vi "nocsac_iface.vi"() -> ()   [LabVIEW 2011]
uses:
  Globals.vi
panel:
  out "Enum":enum16{""}(ring)
  in  "Unlock Door":bool
  out "Door state":bool
  in  "Tab Control":enum32{"Config", "Diag"}(tab)
  in  "Net":bool
  in  "Monitor":i32
  in  "Port":u16
  in  "Node ID":dbl
  out "Conn":bool
  out "remote address":string
  out "remote port":u16
  out "Node ID":u32
  out "Input?":bool
  out "Output?":bool
  out "Psi":bool
  out "Chi":bool
  out "Phi":bool
  out "Upsilon":bool
  out "Omega":bool
  out "Tau":bool
  out "Rho":bool
  out "Pi":bool
  out "Omicron":bool
  out "Xi":bool
  out "Sigma":bool
  out "Nu":bool
  out "Lambda":bool
  out "Kappa":bool
  out "Iota":bool
  out "Theta":bool
  out "Mu":bool
  out "Eta":bool
  out "Epsilon":bool
  out "Delta":bool
  out "Gamma":bool
  out "Beta":bool
  out "Zeta":bool
  out "Alpha":bool
  in  "OMEGA":bool
  in  "PSI":bool
  in  "CHI":bool
  in  "PHI":bool
  in  "UPSILON":bool
  in  "TAU":bool
  in  "SIGMA":bool
  in  "RHO":bool
  in  "PI":bool
  in  "OMICRON":bool
  in  "XI":bool
  in  "NU":bool
  in  "MU":bool
  in  "LAMBDA":bool
  in  "KAPPA":bool
  in  "IOTA":bool
  in  "THETA":bool
  in  "ETA":bool
  in  "ZETA":bool
  in  "EPSILON":bool
  in  "DELTA":bool
  in  "GAMMA":bool
  in  "BETA":bool
  in  "ALPHA":bool
  in  "stop":bool
  in  "Orange":bool
  in  "Chartreuse":bool
  in  "Green":bool
  in  "Fuchsia":bool
  in  "Black":bool
  in  "Grey":bool
  in  "Vermillion":bool
  in  "Beige":bool
  in  "Gold":bool
  in  "Yellow":bool
  in  "Blue":bool
  in  "Red":bool
  out "Red":bool
  out "Orange":bool
  out "Yellow":bool
  out "Green":bool
  out "Vermillion":bool
  out "Orange":bool
  out "Chartreuse":bool
  out "Green":bool
  out "Fuchsia":bool
  out "Black":bool
  out "Grey":bool
  out "Beige":bool
  out "Gold":bool
  out "Yellow":bool
  out "Blue":bool
  out "Red":bool
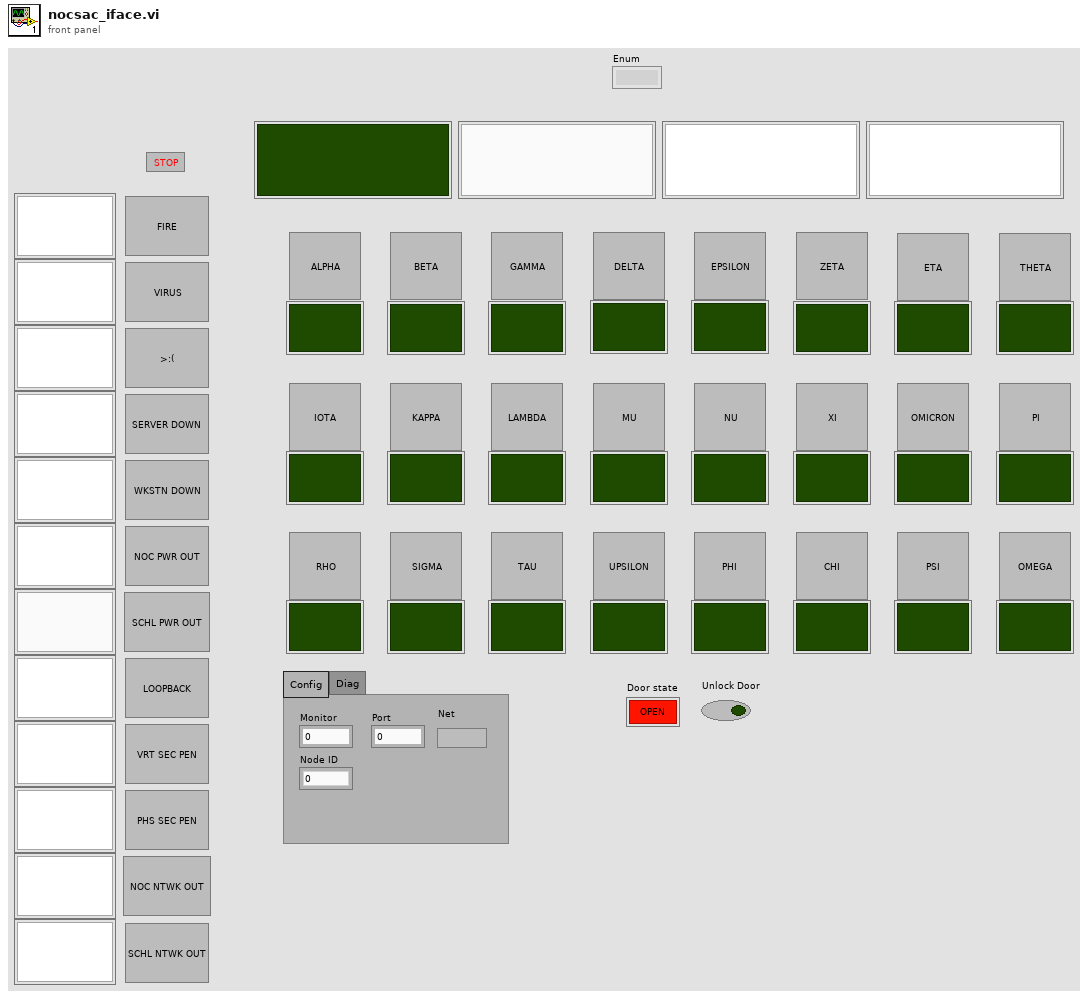
[diagram p1: front panel]
types:
  T1 = typedef "LVAllMonitorsDisplayTypeDef.ctl" = cluster{"Bounds":cluster{"Left":i16, "Top":i16, "Right":i16, "Bottom":i16}, "Depth":i16}[]
  T2 = cluster{"Alpha":bool, "Beta":bool, "Gamma":bool, "Delta":bool, "Epsilon":bool, "Zeta":bool, "Eta":bool, "Theta":bool, "Iota":bool, "Kappa":bool, "Lambda":bool, "Mu":bool, "Nu":bool, "Xi":bool, "Omicron":bool, "Pi":bool, "Rho":bool, "Sigma":bool, "Tau":bool, "Upsilon":bool, "Phi":bool, "Chi":bool, "Psi":bool, "Omega":bool}
  T3 = cluster{"Red":bool, "Blue":bool, "Yellow":bool, "Gold":bool, "Beige":bool, "Grey":bool, "Black":bool, "Fuchsia":bool, "Green":bool, "Chartreuse":bool, "Orange":bool, "Vermillion":bool}
  T4 = cluster{"Bounds":cluster{"Left":i16, "Top":i16, "Right":i16, "Bottom":i16}, "Depth":i16}
  T5 = cluster{"Left":i16, "Top":i16, "Right":i16, "Bottom":i16}
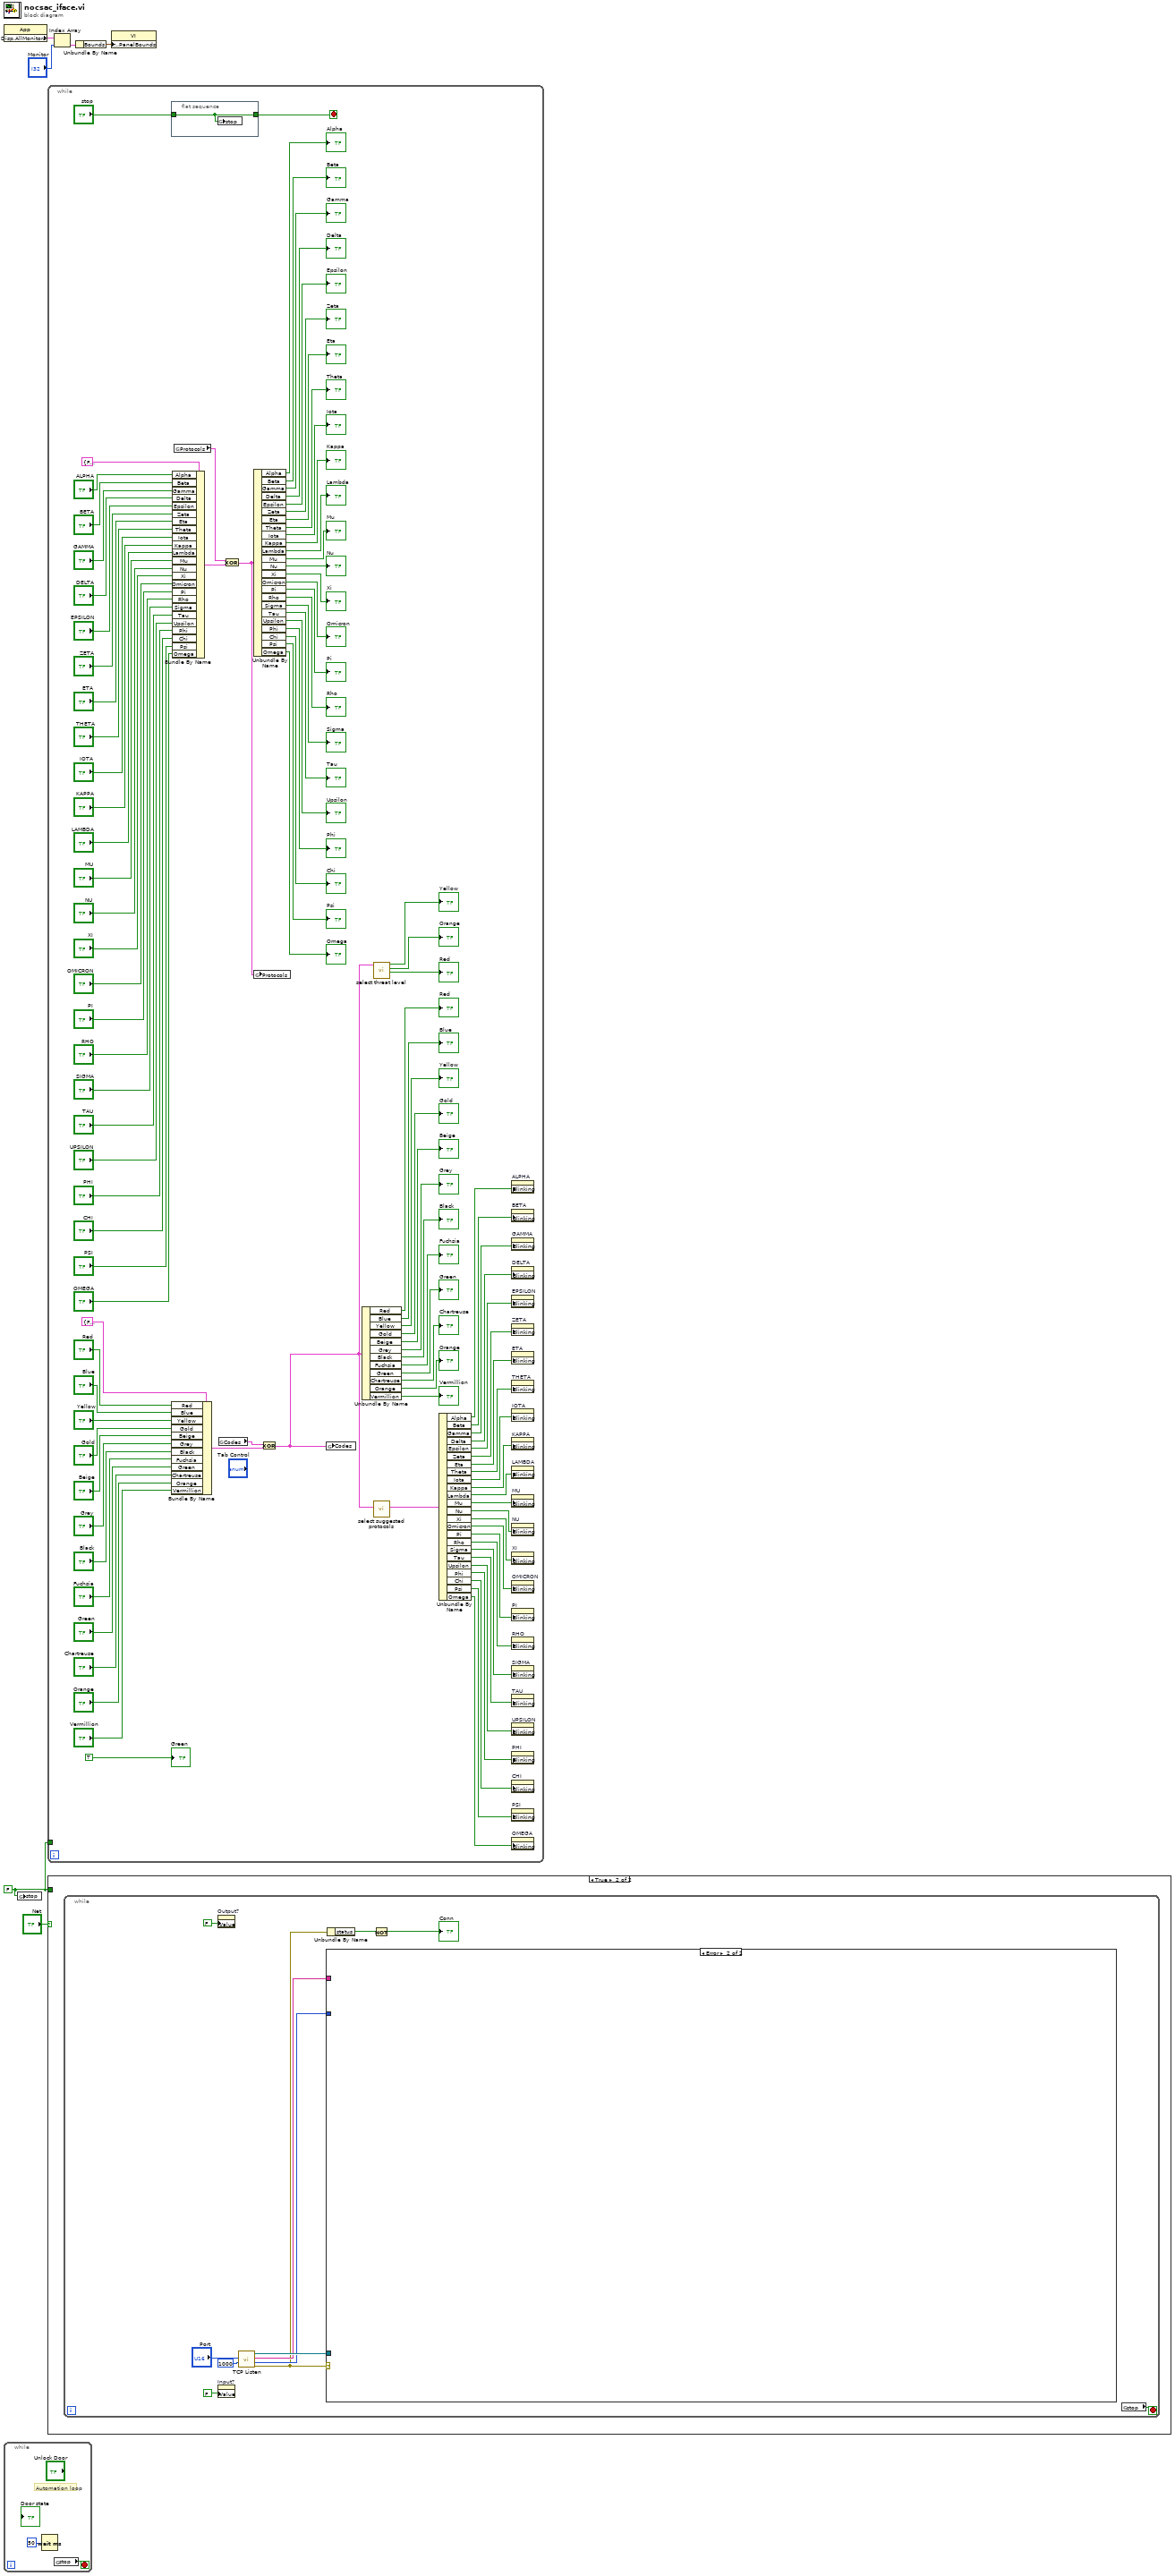
[diagram p0: block diagram]
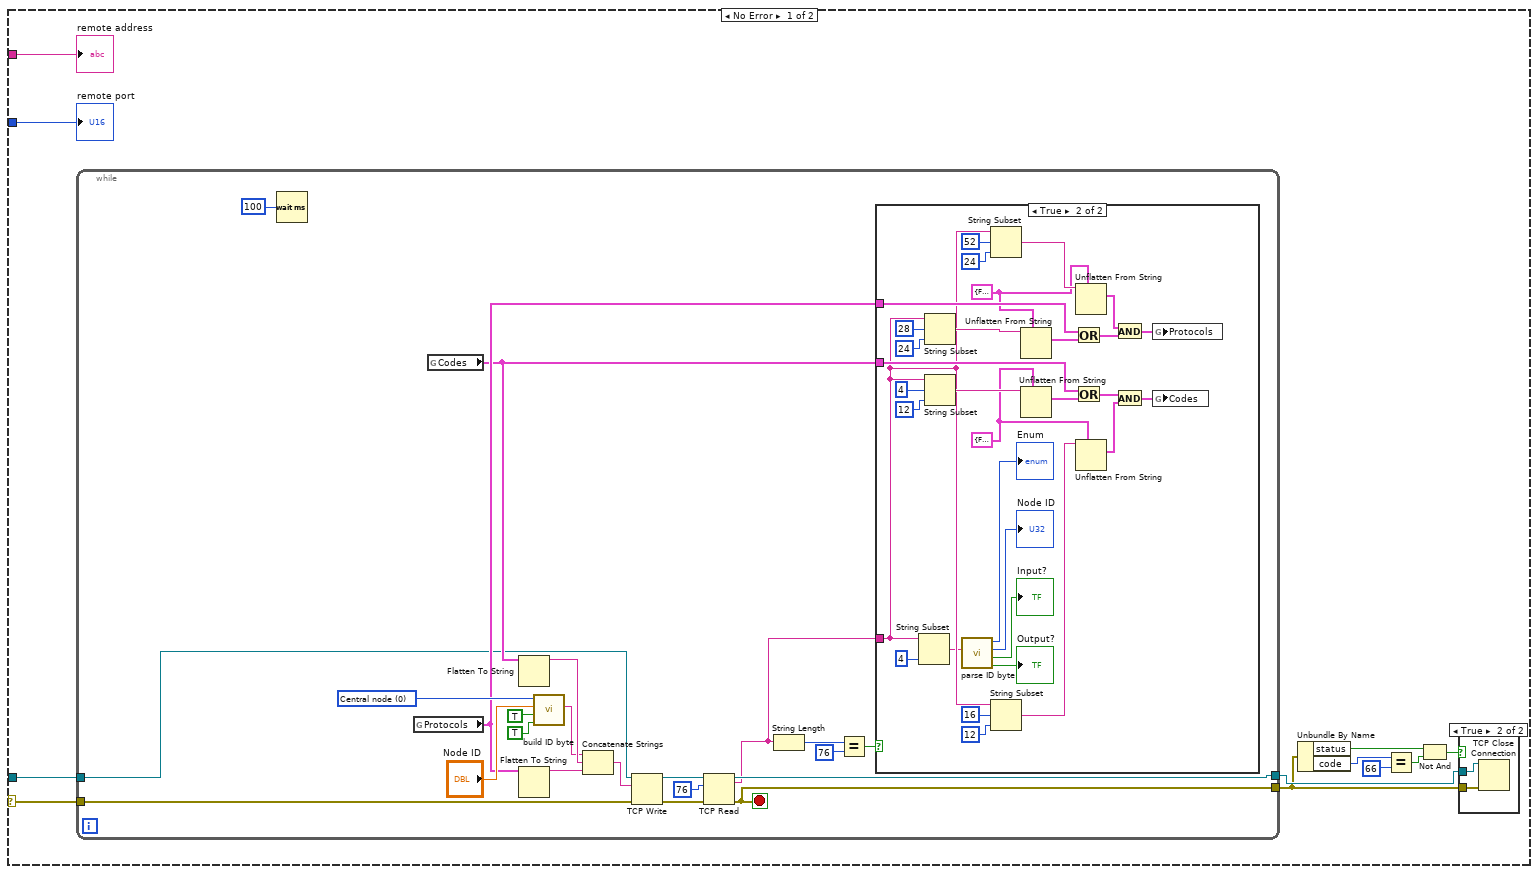
[diagram p3: hidden frame]
diagram:
  w1 = FALSE ("stop")
  n1 = property class="App"() -> ("Disp.AllMonitors"=w6:T1)  [unwired: 2 in, 2 out]
  n2 = while {
    stop <- w7 stop-if-true
    # "Automation loop"
    n3 = Wait (ms)(milliseconds to wait=u32 50) -> ()  [unwired: 1 out]
    n4 = global read "Globals.vi" "stop"() -> (w7:bool)
  }
  n5 = global write "Globals.vi" "stop"(w1) -> ()
  n6 = while {
    tunnel: w1 -> [_]
    stop <- w9 stop-if-true
    n7 = flat-sequence {
      tunnel: "stop" -> [w120]
      tunnel: [w120] -> w9
      frame #0 {
        n8 = global write "Globals.vi" "stop"(w120) -> ()
      }
    }
    n9 = Bundle By Name(cluster=T3 {"Red"=FALSE, "Blue"=FALSE, "Yellow"=FALSE, "Gold"=FALSE, "Beige"=FALSE, "Grey"=FALSE, "Black"=FALSE, "Fuchsia"=FALSE, "Green"=FALSE, "Chartreuse"=FALSE, "Orange"=FALSE, "Vermillion"=FALSE}, "Red"="Red", "Blue"="Blue", "Yellow"="Yellow", "Gold"="Gold", "Beige"="Beige", "Grey"="Grey", "Black"="Black", "Fuchsia"="Fuchsia", "Green"="Green", "Chartreuse"="Chartreuse", "Orange"="Orange", "Vermillion"="Vermillion") -> (w53:T3)
    n10 = Bundle By Name(cluster=T2 {"Alpha"=FALSE, "Beta"=FALSE, "Gamma"=FALSE, "Delta"=FALSE, "Epsilon"=FALSE, "Zeta"=FALSE, "Eta"=FALSE, "Theta"=FALSE, "Iota"=FALSE, "Kappa"=FALSE, "Lambda"=FALSE, "Mu"=FALSE, "Nu"=FALSE, "Xi"=FALSE, "Omicron"=FALSE, "Pi"=FALSE, "Rho"=FALSE, "Sigma"=FALSE, "Tau"=FALSE, "Upsilon"=FALSE, "Phi"=FALSE, "Chi"=FALSE, "Psi"=FALSE, "Omega"=FALSE}, "Alpha"="ALPHA", "Beta"="BETA", "Gamma"="GAMMA", "Delta"="DELTA", "Epsilon"="EPSILON", "Zeta"="ZETA", "Eta"="ETA", "Theta"="THETA", "Iota"="IOTA", "Kappa"="KAPPA", "Lambda"="LAMBDA", "Mu"="MU", "Nu"="NU", "Xi"="XI", "Omicron"="OMICRON", "Pi"="PI", "Rho"="RHO", "Sigma"="SIGMA", "Tau"="TAU", "Upsilon"="UPSILON", "Phi"="PHI", "Chi"="CHI", "Psi"="PSI", "Omega"="OMEGA") -> (w40:T2)
    n11 = global read "Globals.vi" "Protocols"() -> (w38:T2)
    n12 = global read "Globals.vi" "Codes"() -> (w37:T3)
    n13 = Exclusive Or(1:w40, 2:w38) -> (0:w39:T2)
    n14 = Unbundle By Name(w39) -> ("Alpha"=→"Alpha":bool, "Beta"=→"Beta":bool, "Gamma"=→"Gamma":bool, "Delta"=→"Delta":bool, "Epsilon"=→"Epsilon":bool, "Zeta"=→"Zeta":bool, "Eta"=→"Eta":bool, "Theta"=→"Theta":bool, "Iota"=→"Iota":bool, "Kappa"=→"Kappa":bool, "Lambda"=→"Lambda":bool, "Mu"=→"Mu":bool, "Nu"=→"Nu":bool, "Xi"=→"Xi":bool, "Omicron"=→"Omicron":bool, "Pi"=→"Pi":bool, "Rho"=→"Rho":bool, "Sigma"=→"Sigma":bool, "Tau"=→"Tau":bool, "Upsilon"=→"Upsilon":bool, "Phi"=→"Phi":bool, "Chi"=→"Chi":bool, "Psi"=→"Psi":bool, "Omega"=→"Omega":bool)
    n15 = global write "Globals.vi" "Protocols"(w39) -> ()
    n16 = Exclusive Or(1:w53, 2:w37) -> (0:w36:T3)
    n17 = global write "Globals.vi" "Codes"(w36) -> ()
    n18 = Unbundle By Name(w36) -> ("Red"=→"Red":bool, "Blue"=→"Blue":bool, "Yellow"=→"Yellow":bool, "Gold"=→"Gold":bool, "Beige"=→"Beige":bool, "Grey"=→"Grey":bool, "Black"=→"Black":bool, "Fuchsia"=→"Fuchsia":bool, "Green"=→"Green":bool, "Chartreuse"=→"Chartreuse":bool, "Orange"=→"Orange":bool, "Vermillion"=→"Vermillion":bool)
    n19 = call "select threat level.vi"("input cluster"=w36) -> ("Red"=→"Red":bool, "Orange"=→"Orange":bool, "Yellow"=→"Yellow":bool)  [unwired: 8 in]
    n20 = call "select suggested protocols.vi"("Codes"=w36) -> ("To blink PN's"=w35:T2)  [unwired: 10 in]
    n21 = Unbundle By Name(w35) -> ("Alpha"=w20:bool, "Beta"=w11:bool, "Gamma"=w33:bool, "Delta"=w31:bool, "Epsilon"=w28:bool, "Zeta"=w12:bool, "Eta"=w27:bool, "Theta"=w13:bool, "Iota"=w26:bool, "Kappa"=w29:bool, "Lambda"=w14:bool, "Mu"=w21:bool, "Nu"=w18:bool, "Xi"=w24:bool, "Omicron"=w34:bool, "Pi"=w23:bool, "Rho"=w19:bool, "Sigma"=w25:bool, "Tau"=w22:bool, "Upsilon"=w16:bool, "Phi"=w32:bool, "Chi"=w30:bool, "Psi"=w17:bool, "Omega"=w15:bool)
    n22 = property on="ALPHA" class="Bool"("Blinking"=w20) -> ()  [unwired: 2 in, 2 out]
    n23 = property on="BETA" class="Bool"("Blinking"=w11) -> ()  [unwired: 2 in, 2 out]
    n24 = property on="GAMMA" class="Bool"("Blinking"=w33) -> ()  [unwired: 2 in, 2 out]
    n25 = property on="DELTA" class="Bool"("Blinking"=w31) -> ()  [unwired: 2 in, 2 out]
    n26 = property on="EPSILON" class="Bool"("Blinking"=w28) -> ()  [unwired: 2 in, 2 out]
    n27 = property on="ZETA" class="Bool"("Blinking"=w12) -> ()  [unwired: 2 in, 2 out]
    n28 = property on="ETA" class="Bool"("Blinking"=w27) -> ()  [unwired: 2 in, 2 out]
    n29 = property on="THETA" class="Bool"("Blinking"=w13) -> ()  [unwired: 2 in, 2 out]
    n30 = property on="IOTA" class="Bool"("Blinking"=w26) -> ()  [unwired: 2 in, 2 out]
    n31 = property on="KAPPA" class="Bool"("Blinking"=w29) -> ()  [unwired: 2 in, 2 out]
    n32 = property on="LAMBDA" class="Bool"("Blinking"=w14) -> ()  [unwired: 2 in, 2 out]
    n33 = property on="MU" class="Bool"("Blinking"=w21) -> ()  [unwired: 2 in, 2 out]
    n34 = property on="NU" class="Bool"("Blinking"=w18) -> ()  [unwired: 2 in, 2 out]
    n35 = property on="XI" class="Bool"("Blinking"=w24) -> ()  [unwired: 2 in, 2 out]
    n36 = property on="OMICRON" class="Bool"("Blinking"=w34) -> ()  [unwired: 2 in, 2 out]
    n37 = property on="PI" class="Bool"("Blinking"=w23) -> ()  [unwired: 2 in, 2 out]
    n38 = property on="RHO" class="Bool"("Blinking"=w19) -> ()  [unwired: 2 in, 2 out]
    n39 = property on="SIGMA" class="Bool"("Blinking"=w25) -> ()  [unwired: 2 in, 2 out]
    n40 = property on="TAU" class="Bool"("Blinking"=w22) -> ()  [unwired: 2 in, 2 out]
    n41 = property on="UPSILON" class="Bool"("Blinking"=w16) -> ()  [unwired: 2 in, 2 out]
    n42 = property on="PHI" class="Bool"("Blinking"=w32) -> ()  [unwired: 2 in, 2 out]
    n43 = property on="CHI" class="Bool"("Blinking"=w30) -> ()  [unwired: 2 in, 2 out]
    n44 = property on="PSI" class="Bool"("Blinking"=w17) -> ()  [unwired: 2 in, 2 out]
    n45 = property on="OMEGA" class="Bool"("Blinking"=w15) -> ()  [unwired: 2 in, 2 out]
    "Green" <- TRUE ("Green")
  }
  n46 = case shown="True" "Net" {
    tunnel: w1 -> [_ _]
    frame False {
    }
    frame True {
      n47 = while {
        stop <- w129 stop-if-true
        n48 = property on="Output?" class="Bool (strict)"("Value"=FALSE ("Output?")) -> ()  [unwired: 2 in, 2 out]
        n49 = property on="Input?" class="Bool (strict)"("Value"=FALSE ("Input?")) -> ()  [unwired: 2 in, 2 out]
        n50 = call <vilib>:"TCP Listen.vi"("timeout ms (wait forever: -1)"=1000, "port"="Port") -> ("error out"=w125:errorcluster, "remote port"=w126:u16, "remote address"=w127:string, "connection ID"=w131:refnum<k5>)  [unwired: 5 in, 1 out]
        n51 = case shown="Error" w125 {
          selector: w125 -> [w140 _]
          tunnel: w131 -> [w142 _]
          tunnel: w127 -> [w139 _]
          tunnel: w126 -> [w138 _]
          frame No Error {
            n52 = while {
              tunnel: w142 -> [w155]
              tunnel: w140 -> [w147]
              tunnel: [w145] -> w137
              tunnel: [w159] -> w141
              stop <- w145 stop-if-true
              w166 = u16 0 items=["Central node", "Portable control", "Boolean sensor", "Boolean output", "8-bit sensor", "8-bit output"] ("Type")
              n53 = Wait (ms)(milliseconds to wait=u32 100) -> ()  [unwired: 1 out]
              n54 = global read "Globals.vi" "Protocols"() -> (w158:T2)
              n55 = global read "Globals.vi" "Codes"() -> (w156:T3)
              n56 = Flatten To String(anything=w156) -> (data string=w154:string)  [unwired: 3 in, 2 out]
              n57 = Flatten To String(anything=w158) -> (data string=w163:string)  [unwired: 3 in, 2 out]
              n58 = call "build ID byte.vi"("Output?"=TRUE, "Input?"=TRUE, "Node ID"="Node ID", "Type"=w166) -> ("ID byte"=w152:string)  [unwired: 6 in, 1 out]
              n59 = Concatenate Strings(w152, w154, w163) -> (w153:string)
              n60 = TCP Write(connection ID=w155, data in=w153, error in (no error)=w147) -> (connection ID out=w160:refnum<k5>, error out=w161:errorcluster)  [unwired: 1 in, 1 out]
              n61 = TCP Read(connection ID=w160, bytes to read=76, error in (no error)=w161) -> (connection ID out=w159:refnum<k5>, data out=w150:string, error out=w145:errorcluster)  [unwired: 2 in]
              n62 = String Length(string=w150) -> (length=w149:i32)
              n63 = Equal?(x=w149, y=76) -> (x = y?=w146:bool)
              n64 = case shown="True" w146 {
                tunnel: w158 -> [_ w197]
                tunnel: w156 -> [_ w196]
                tunnel: w150 -> [_ w173]
                frame False {
                }
                frame True {
                  w177 = T2 {"Alpha"=FALSE, "Beta"=FALSE, "Gamma"=FALSE, "Delta"=FALSE, "Epsilon"=FALSE, "Zeta"=FALSE, "Eta"=FALSE, "Theta"=FALSE, "Iota"=FALSE, "Kappa"=FALSE, "Lambda"=FALSE, "Mu"=FALSE, "Nu"=FALSE, "Xi"=FALSE, "Omicron"=FALSE, "Pi"=FALSE, "Rho"=FALSE, "Sigma"=FALSE, "Tau"=FALSE, "Upsilon"=FALSE, "Phi"=FALSE, "Chi"=FALSE, "Psi"=FALSE, "Omega"=FALSE}
                  w189 = T3 {"Red"=FALSE, "Blue"=FALSE, "Yellow"=FALSE, "Gold"=FALSE, "Beige"=FALSE, "Grey"=FALSE, "Black"=FALSE, "Fuchsia"=FALSE, "Green"=FALSE, "Chartreuse"=FALSE, "Orange"=FALSE, "Vermillion"=FALSE}
                  n65 = String Subset(string=w173, length (rest)=4 ("length (rest)")) -> (substring=w171:string)  [unwired: 1 in]
                  n66 = String Subset(string=w173, offset (0)=28, length (rest)=24 ("length (rest)")) -> (substring=w182:string)
                  n67 = String Subset(string=w173, offset (0)=4, length (rest)=12 ("length (rest)")) -> (substring=w191:string)
                  n68 = call "parse ID byte.vi"("ID byte"=w171) -> ("Output?"=→"Output?":bool, "Input?"=→"Input?":bool, "Node ID"=→"Node ID":u32, "Enum"=→"Enum":enum16{""})  [unwired: 7 in]
                  n69 = String Subset(string=w173, offset (0)=52, length (rest)=24 ("length (rest)")) -> (substring=w178:string)
                  n70 = String Subset(string=w173, offset (0)=16, length (rest)=12 ("length (rest)")) -> (substring=w190:string)
                  n71 = Unflatten From String(type=w177, binary string=w182) -> (value=w181:T2)  [unwired: 3 in, 2 out]
                  n72 = Unflatten From String(type=w189, binary string=w191) -> (value=w185:T3)  [unwired: 3 in, 2 out]
                  n73 = Or(x=w197, y=w181) -> (x .or. y?=w175:T2)
                  n74 = Or(x=w196, y=w185) -> (x .or. y?=w188:T3)
                  n75 = Unflatten From String(type=w177, binary string=w178) -> (value=w176:T2)  [unwired: 3 in, 2 out]
                  n76 = Unflatten From String(type=w189, binary string=w190) -> (value=w187:T3)  [unwired: 3 in, 2 out]
                  n77 = And(x=w176, y=w175) -> (x .and. y?=w174:T2)
                  n78 = And(x=w188, y=w187) -> (x .and. y?=w186:T3)
                  n79 = global write "Globals.vi" "Protocols"(w174) -> ()
                  n80 = global write "Globals.vi" "Codes"(w186) -> ()
                }
              }
            }
            n81 = Unbundle By Name(w137) -> ("status"=w133:bool, "code"=w136:i32)
            n82 = Equal?(x=w136, y=66) -> (x = y?=w132:bool)
            n83 = Not And(1:w132, 2:w133) -> (0:w134:bool)
            n84 = case shown="True" w134 {
              tunnel: w141 -> [_ w144]
              tunnel: w137 -> [_ w143]
              frame False {
              }
              frame True {
                n85 = TCP Close Connection(connection ID=w144, error in (no error)=w143) -> ()  [unwired: 1 in, 2 out]
              }
            }
            "remote address" <- w139
            "remote port" <- w138
          }
          frame Error {
          }
        }
        n86 = Unbundle By Name(w125) -> ("status"=w123:bool)
        n87 = Not(x=w123) -> (.not. x?=→"Conn":bool)
        n88 = global read "Globals.vi" "stop"() -> (w129:bool)
      }
    }
  }
  n89 = Index Array(array=w6, index="Monitor") -> (element=w5:T4)
  n90 = Unbundle By Name(w5) -> ("Bounds"=w4:T5)
  n91 = property class="VI"("Front Panel.PanelBounds"=w4) -> ()  [unwired: 2 in, 2 out]
